vi "OAT Detrend Analog Tacho Signal.vi"   [LabVIEW 2017, in "SoundVib_TachProcess.lvlib"]
doc: "Removes trend from an analog tachometer signal. You can use the output of this VI as an input for the OAT Analog Tacho Process VI. Wire data to the <B>analog tacho signal</B> input to determine the polymorphic instance to use or manually select the instance."
uses:
  <vilib>/addons/Sound and Vibration/Order Analysis/Tach Process/SoundVib_TachProcess.lvlib
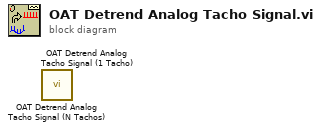
[diagram p0: block diagram]
diagram:
  n1 = call <vilib>:"OAT Detrend Analog Tacho Signal (N Tachos).vi"() -> ()  [unwired: 13 in, 3 out]
  n2 = call <vilib>:"OAT Detrend Analog Tacho Signal (1 Tacho).vi"() -> ()  [unwired: 13 in, 3 out]
